vi "Sim_Main.vi"(1 "Motor Voltages":cluster{"Left Voltage":dbl, "Right Voltage":dbl}, 2 "Input Telemetry":T1) -> (0 "Output Telemetry":T1)   [LabVIEW 2009]
panel:
  in  "Inertia":dbl=0.02
  in  "Mass":dbl=1.0
  in  "Delta t":dbl=0.01
  in  "Left Voltage":dbl
  in  "Right Voltage":dbl
  out "Right Thrust":dbl
  out "Left Thrust":dbl
  out "Theta":dbl
  out "Omega":dbl
  out "Alpha":dbl
  out "Ay":dbl
  out "Ax":dbl
  out "Vy":dbl
  out "Y":dbl
  out "Vx":dbl
  out "X":dbl
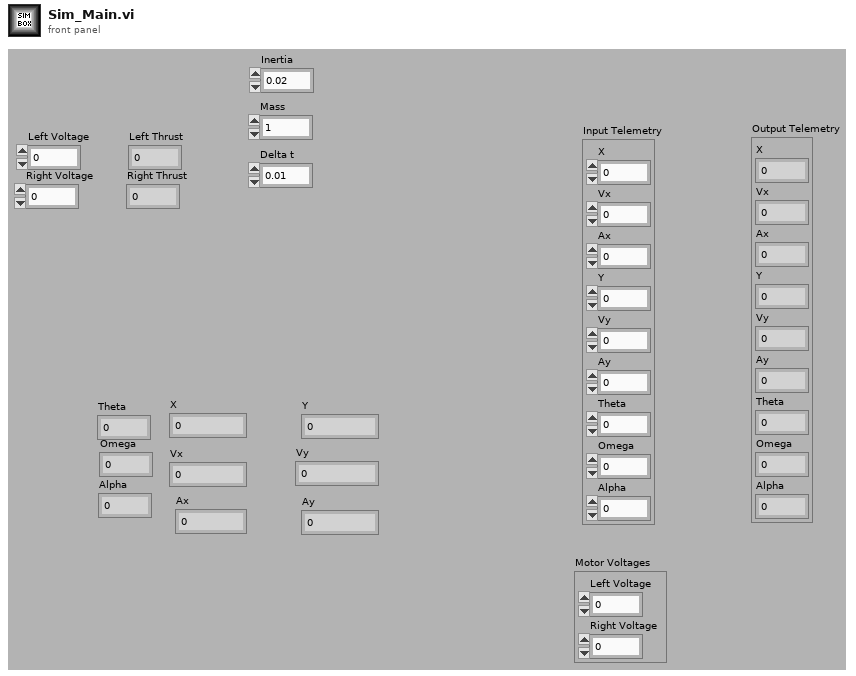
[diagram p1: front panel]
types:
  T1 = cluster{"X":dbl, "Vx":dbl, "Ax":dbl, "Y":dbl, "Vy":dbl, "Ay":dbl, "Theta":dbl, "Omega":dbl, "Alpha":dbl}
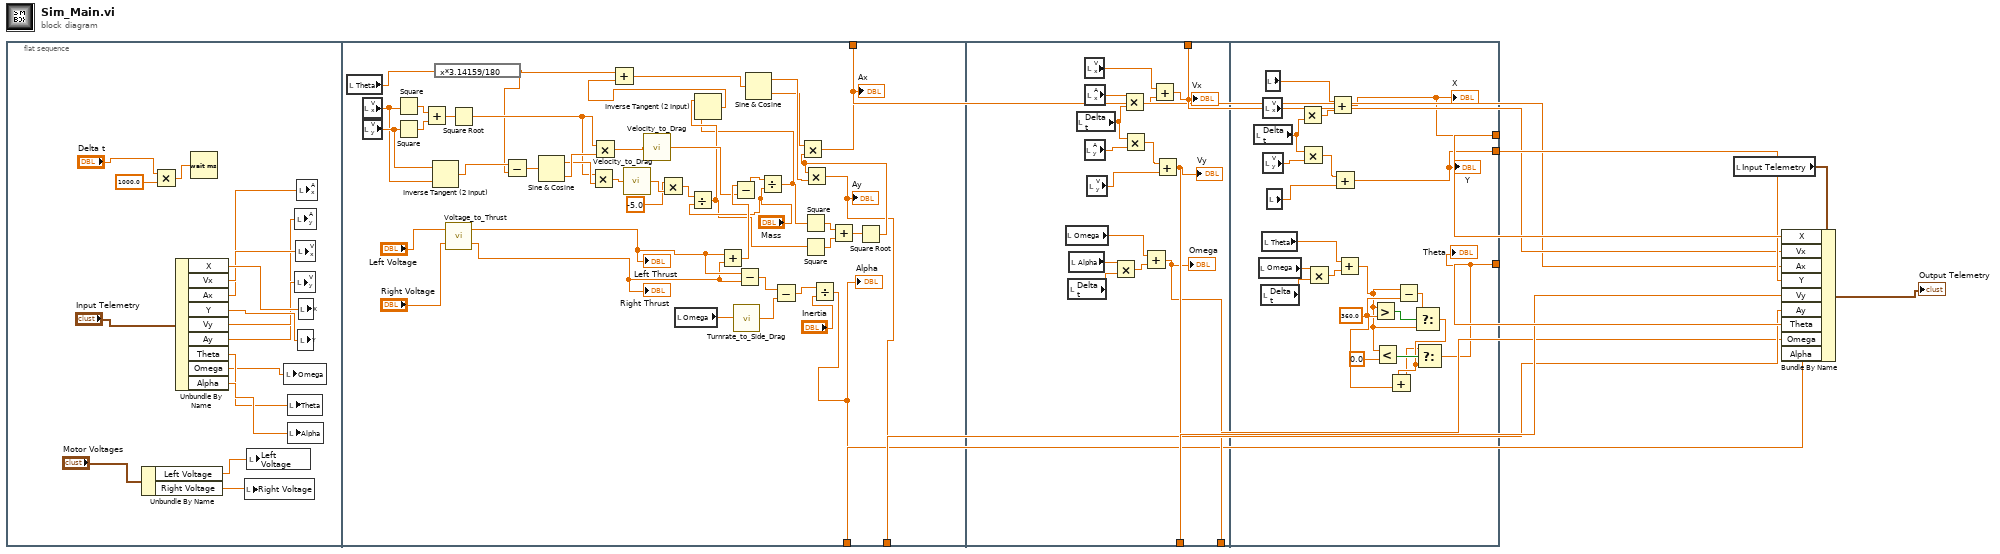
[diagram p0: block diagram]
diagram:
  n1 = flat-sequence {
    tunnel: [w31] -> w4
    tunnel: [w30] -> w3
    tunnel: [w29] -> w1
    tunnel: [w73] -> w6
    tunnel: [w72] -> w5
    tunnel: [w71] -> w2
    tunnel: [w99] -> w9
    tunnel: [w98] -> w8
    tunnel: [w85] -> w7
    frame #0 {
      n2 = Unbundle By Name("Motor Voltages") -> ("Left Voltage"=w22:dbl, "Right Voltage"=w23:dbl)
      n3 = Multiply(x="Delta t", y=1000.0) -> (x*y=w24:dbl)
      n4 = Unbundle By Name("Input Telemetry") -> ("X"=w16:dbl, "Vx"=w15:dbl, "Ax"=w12:dbl, "Y"=w17:dbl, "Vy"=w14:dbl, "Ay"=w13:dbl, "Theta"=w19:dbl, "Omega"=w18:dbl, "Alpha"=w20:dbl)
      n5 = Wait (ms)(milliseconds to wait=w24) -> ()  [unwired: 1 out]
      n6 = local write "Right Voltage"(w23) -> ()
      n7 = local write "Left Voltage"(w22) -> ()
      n8 = local write "Omega"(w18) -> ()
      n9 = local write "Theta"(w19) -> ()
      n10 = local write "Alpha"(w20) -> ()
      n11 = local write "Ay"(w13) -> ()
      n12 = local write "Vy"(w14) -> ()
      n13 = local write "Vx"(w15) -> ()
      n14 = local write "Ax"(w12) -> ()
      n15 = local write "Y"(w17) -> ()
      n16 = local write "X"(w16) -> ()
    }
    frame #1 {
      n17 = local read "Theta"() -> (w28:dbl)
      n18 = local read "Vx"() -> (w58:dbl)
      n19 = local read "Vy"() -> (w59:dbl)
      n20 = Square(x=w58) -> (x^2=w69:dbl)
      n21 = Square(x=w59) -> (x^2=w68:dbl)
      n22 = Add(x=w69, y=w68) -> (x+y=w67:dbl)
      n23 = Inverse Tangent (2 Input)(1:w58, 2:w59) -> (0:w57:dbl)
      n24 = expression code="x*3.14159/180"(w28) -> (w40:dbl)
      n25 = call "Voltage_to_Thrust.vi"("Right Voltage"="Right Voltage", "Left Voltage"="Left Voltage") -> ("Right Thrust"=w32:dbl, "Left Thrust"=w33:dbl)
      "Left Thrust" <- w33
      "Right Thrust" <- w32
      n26 = Square Root(x=w67) -> (sqrt(x)=w52:dbl)
      n27 = Subtract(x=w57, y=w40) -> (x-y=w56:dbl)
      n28 = Sine & Cosine(0:w56) -> (1:w53:dbl, 2:w55:dbl)
      n29 = Multiply(x=w52, y=w53) -> (x*y=w51:dbl)
      n30 = Multiply(x=w52, y=w55) -> (x*y=w54:dbl)
      n31 = call "Velocity_to_Drag.vi"("Velocity"=w51) -> ("Drag"=w50:dbl)
      n32 = call "Velocity_to_Drag.vi"("Velocity"=w54) -> ("Drag"=w65:dbl)
      n33 = Multiply(x=-5.0, y=w50) -> (x*y=w48:dbl)
      n34 = local read "Omega"() -> (w70:dbl)
      n35 = Divide(x=w48, y="Mass") -> (x/y=w42:dbl)
      n36 = Add(x=w33, y=w32) -> (x+y=w66:dbl)
      n37 = Subtract(x=w66, y=w65) -> (x-y=w64:dbl)
      n38 = call "Turnrate_to_Side_Drag.vi"("Turn Rate"=w70) -> ("Side Drag"=w62:dbl)
      n39 = Subtract(x=w33, y=w32) -> (x-y=w63:dbl)
      n40 = Divide(x=w64, y="Mass") -> (x/y=w41:dbl)
      n41 = Inverse Tangent (2 Input)(1:w41, 2:w42) -> (0:w39:dbl)
      n42 = Add(x=w40, y=w39) -> (x+y=w38:dbl)
      n43 = Sine & Cosine(0:w38) -> (1:w37:dbl, 2:w36:dbl)
      n44 = Subtract(x=w63, y=w62) -> (x-y=w61:dbl)
      n45 = Square(x=w41) -> (x^2=w44:dbl)
      n46 = Square(x=w42) -> (x^2=w45:dbl)
      n47 = Divide(x=w61, y="Inertia") -> (x/y=w29:dbl)
      "Alpha" <- w29
      n48 = Add(x=w44, y=w45) -> (x+y=w46:dbl)
      n49 = Square Root(x=w46) -> (sqrt(x)=w43:dbl)
      n50 = Multiply(x=w36, y=w43) -> (x*y=w31:dbl)
      "Ax" <- w31
      n51 = Multiply(x=w43, y=w37) -> (x*y=w30:dbl)
      "Ay" <- w30
    }
    frame #2 {
      n52 = local read "Omega"() -> (w76:dbl)
      n53 = local read "Delta t"() -> (w77:dbl)
      n54 = local read "Alpha"() -> (w74:dbl)
      n55 = local read "Delta t"() -> (w80:dbl)
      n56 = local read "Ay"() -> (w81:dbl)
      n57 = local read "Vx"() -> (w82:dbl)
      n58 = local read "Ax"() -> (w84:dbl)
      n59 = local read "Vy"() -> (w78:dbl)
      n60 = Multiply(x=w74, y=w77) -> (x*y=w75:dbl)
      n61 = Multiply(x=w84, y=w80) -> (x*y=w83:dbl)
      n62 = Multiply(x=w80, y=w81) -> (x*y=w79:dbl)
      n63 = Add(x=w76, y=w75) -> (x+y=w71:dbl)
      "Omega" <- w71
      n64 = Add(x=w82, y=w83) -> (x+y=w73:dbl)
      "Vx" <- w73
      n65 = Add(x=w79, y=w78) -> (x+y=w72:dbl)
      "Vy" <- w72
    }
    frame #3 {
      w87 = 360.0 ("y")
      n66 = local read "Delta t"() -> (w104:dbl)
      n67 = local read "Omega"() -> (w97:dbl)
      n68 = local read "Delta t"() -> (w94:dbl)
      n69 = local read "Theta"() -> (w95:dbl)
      n70 = local read "Vx"() -> (w100:dbl)
      n71 = local read "Vy"() -> (w103:dbl)
      n72 = local read "X"() -> (w102:dbl)
      n73 = local read "Y"() -> (w106:dbl)
      n74 = Multiply(x=w100, y=w104) -> (x*y=w101:dbl)
      n75 = Multiply(x=w104, y=w103) -> (x*y=w105:dbl)
      n76 = Multiply(x=w97, y=w94) -> (x*y=w96:dbl)
      n77 = Add(x=w102, y=w101) -> (x+y=w99:dbl)
      "X" <- w99
      n78 = Add(x=w105, y=w106) -> (x+y=w98:dbl)
      "Y" <- w98
      n79 = Add(x=w95, y=w96) -> (x+y=w86:dbl)
      n80 = Greater?(x=w86, y=w87) -> (0:w92:bool)
      n81 = Less?(x=w86, y=0.0) -> (x < y?=w91:bool)
      n82 = Subtract(x=w86, y=w87) -> (x-y=w88:dbl)
      n83 = Select(t=w88, s=w92, f=w86) -> (s? t:f=w90:dbl)
      n84 = Add(x=w90, y=w87) -> (x+y=w89:dbl)
      n85 = Select(t=w89, s=w91, f=w90) -> (s? t:f=w85:dbl)
      "Theta" <- w85
    }
  }
  n86 = local read "Input Telemetry"() -> (w11:T1)
  n87 = Bundle By Name(cluster=w11, "X"=w9, "Vx"=w6, "Ax"=w4, "Y"=w8, "Vy"=w5, "Ay"=w3, "Theta"=w7, "Omega"=w2, "Alpha"=w1) -> (→"Output Telemetry":T1)
